vi "Case structures1.vi"() -> ()   [LabVIEW 2024]
panel:
  in  "Boolean":bool
  out "x-y":dbl
  out "Add res":dbl
  in  "Y":dbl
  in  "x":i32
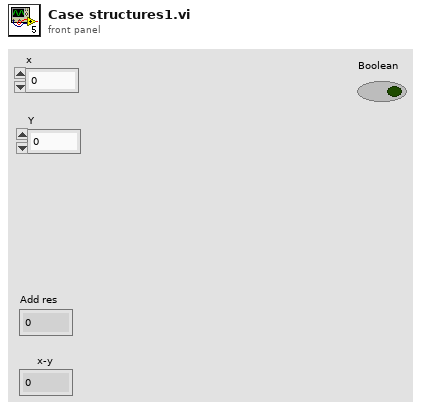
[diagram p1: front panel]
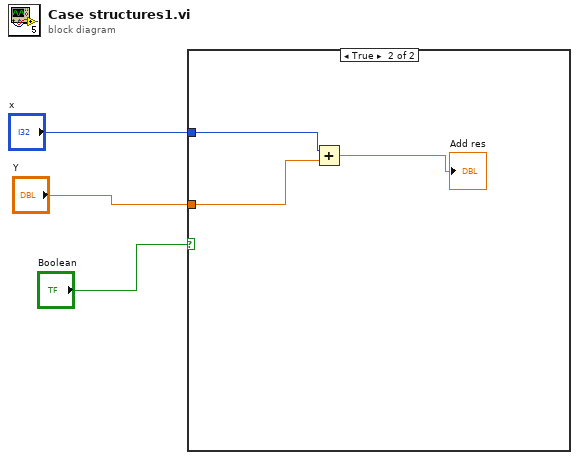
[diagram p0: block diagram]
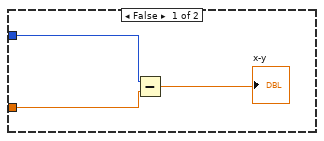
[diagram p2: hidden frame]
diagram:
  n1 = case shown="True" "Boolean" {
    tunnel: "x" -> [w6 w9]
    tunnel: "Y" -> [w5 w8]
    frame False {
      n2 = Subtract(x=w6, y=w5) -> (x-y=→"x-y":dbl)
    }
    frame True {
      n3 = Add(x=w9, y=w8) -> (x+y=→"Add res":dbl)
    }
  }
